vi "监测浓度升序排列 (子VI).vi"(9 "标液浓度":dbl[](array[numeric]), 10 "滴定数":dbl[](array[numeric]), 11 "启用":bool[](array[boolean])) -> (3 "输出数组":dbl[][](array[numeric]))   [LabVIEW 2016, in "斯坦道原位多参数.lvlib"]
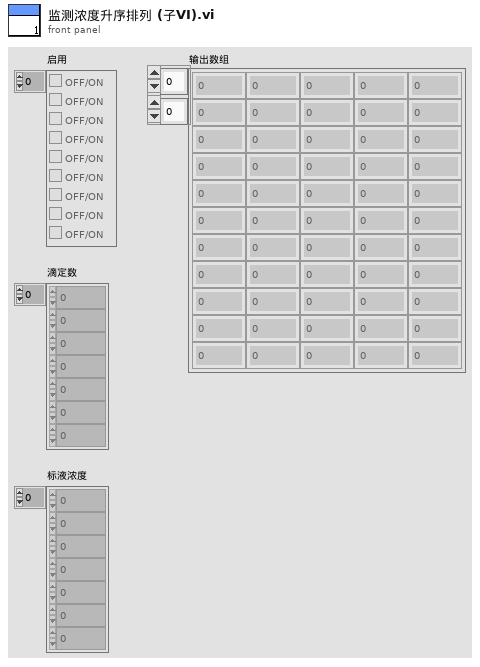
[diagram p1: front panel]
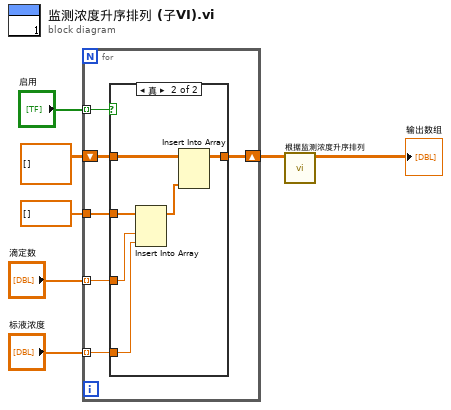
[diagram p0: block diagram]
diagram:
  n1 = for {
    tunnel: "启用" -> [w8] mode=indexing
    tunnel: "滴定数" -> [w11] mode=indexing
    tunnel: "标液浓度" -> [w10] mode=indexing
    shift-right: [w9] -> w7
    shift-left: dbl[][] [] ("标液浓度") -> [w13]
    tunnel: dbl[] [] ("监测浓度") -> [w12]
    n2 = case shown="真" w8 {
      tunnel: w13 -> [w14 w20]
      tunnel: w12 -> [_ w19]
      tunnel: w11 -> [_ w18]
      tunnel: w10 -> [_ w17]
      tunnel: [w14 w15] -> w9
      frame False {
      }
      frame True {
        n3 = Insert Into Array(array=w19, new element #1=w18, new element #2=w17) -> (w16:dbl[])  [unwired: 1 in]
        n4 = Insert Into Array(array=w20, new element=w16) -> (w15:dbl[][])  [unwired: 2 in]
      }
    }
  }
  n5 = call "根据监测浓度升序排列.vi"("标液浓度输入"=w7) -> ("输出数组"=→"输出数组":dbl[][])  [unwired: 10 in]
